vi "Create File for Drive SS.vi"() -> (2 "File Reference Out":refnum<file>)   [LabVIEW 2016]
uses:
  Global Variables/Folder Names.vi
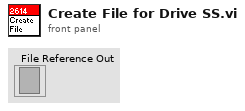
[diagram p1: front panel]
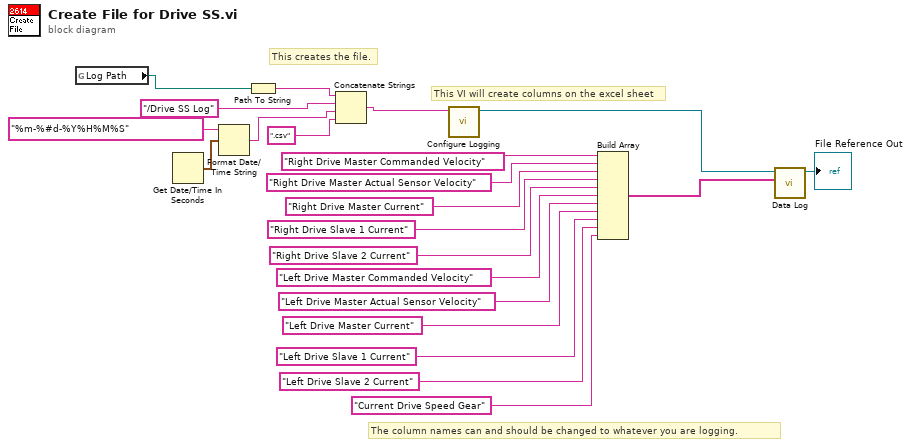
[diagram p0: block diagram]
diagram:
  # "The column names can and should be changed to whatever you are logging."
  # "This VI will create columns on the excel sheet"
  # "This creates the file."
  n1 = global read "Folder Names.vi" "Log Path"() -> (w20:path)
  n2 = Get Date/Time In Seconds() -> (seconds since 1Jan1904=w11:timestamp)
  n3 = Format Date/Time String(time format string (%c)="%m-%#d-%Y%H%M%S", seconds (now)=w11) -> (date/time string=w9:string)  [unwired: 1 in]
  n4 = Path To String(path=w20) -> (string=w19:string)
  n5 = Concatenate Strings(w19, "/Drive SS Log" ("string"), w9, ".csv" ("string")) -> (w21:string)
  n6 = call "Configure Logging.vi"("File Path/File Name"=w21) -> ("refnum out"=w13:refnum<file>)  [unwired: 10 in]
  n7 = Build Array("Right Drive Master Commanded Velocity" ("File Path/File Name"), "Right Drive Master Actual Sensor Velocity" ("File Path/File Name"), "Right Drive Master Current", "Right Drive Slave 1 Current", "Right Drive Slave 2 Current", "Left Drive Master Commanded Velocity" ("File Path/File Name"), "Left Drive Master Actual Sensor Velocity" ("File Path/File Name"), "Left Drive Master Current", "Left Drive Slave 1 Current", "Left Drive Slave 2 Current", "Current Drive Speed Gear" ("File Path/File Name")) -> (w18:string[])
  n8 = call "Data Log.vi"("Data In"=w18, "File Reference In"=w13) -> ("File Reference Out"=→"File Reference Out":refnum<file>)  [unwired: 9 in]
